vi "CameraReadJPEG.vi"(11 "IO Cluster In":T1={"Error"={"status"=FALSE, "code"=0, "source"=""}, "Encoder Calibration Values"=[22, 216], "Update Calibration"=FALSE, "JPEG Resolutions"=3, "Raw Resolutions"=1, "Image Mode"=enum."RAW Gray Scale", "FPGA Ref"=refnum} {"JPEG Resolutions" items=["160x128"=3, "320x240"=5, "640x480"=7]; "Raw Resolutions" items=["80x60"=1, "160x120"=3, "128x128"=9, "128x96"=11]}) -> (1 "New Image Data":bool, 2 "Image Data":u8[](array[numeric]) format="%02x", 3 "IO Cluster Out":T1={"Error"={"status"=FALSE, "code"=0, "source"=""}, "Encoder Calibration Values"=[22, 216], "Update Calibration"=FALSE, "JPEG Resolutions"=3, "Raw Resolutions"=1, "Image Mode"=enum."RAW Gray Scale", "FPGA Ref"=refnum} {"JPEG Resolutions" items=["160x128"=3, "320x240"=5, "640x480"=7]; "Raw Resolutions" items=["80x60"=1, "160x120"=3, "128x128"=9, "128x96"=11]}, 4 "Bytes in Buffer":u32, 5 "Image Comm Error":bool)   [LabVIEW 2019]
uses:
  JPEG Read States.ctl
  QNET MS IO Cluster.ctl
panel:
  out "Current Package":u16
  out "Picture Info Bytes":u8[](array[numeric]) format="%x"
  out "Packages":u32
  out "State":T2=enum."JPEG Picture Info"
  out "Wait for Get Picture ACK Error":bool
  out "Raw Picture Info Error":bool
  out "Bytes to Recieve":u32
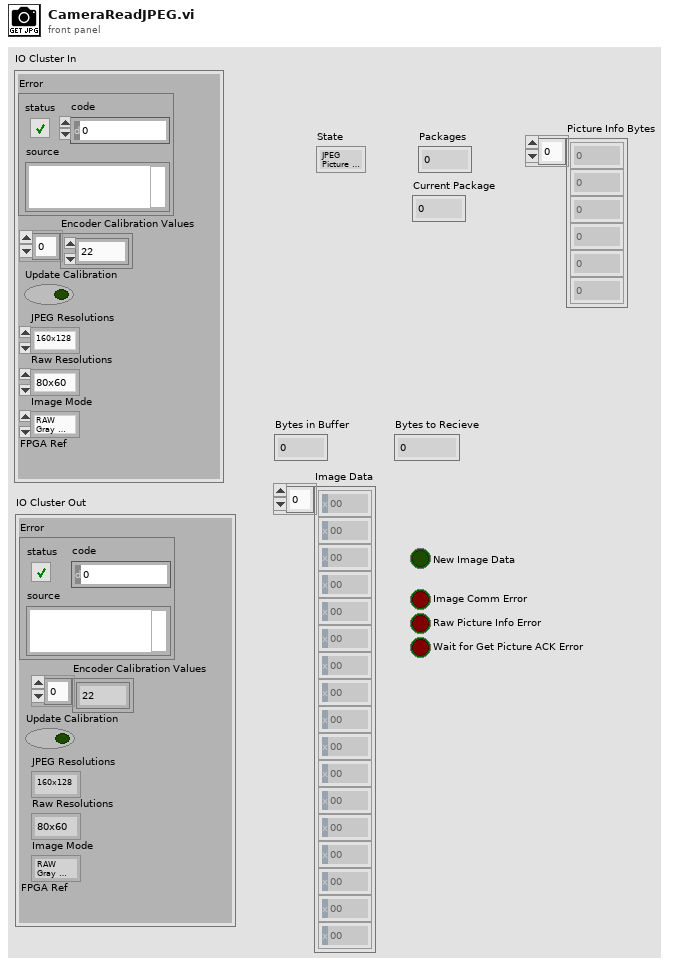
[diagram p1: front panel]
types:
  T1 = typedef "QNET MS IO Cluster.ctl" = cluster{"Error":errorcluster, "Encoder Calibration Values":i32[], "Update Calibration":bool, "JPEG Resolutions":u16, "Raw Resolutions":u16, "Image Mode":enum16{"RAW RGB", "RAW Gray Scale", "JPEG"}, "FPGA Ref":refnum<k20>}
  T2 = typedef "JPEG Read States.ctl" = enum16{"Wait for ACK", "Request Picture", "JPEG Picture Info", "Done", "Error", "Image Data"}
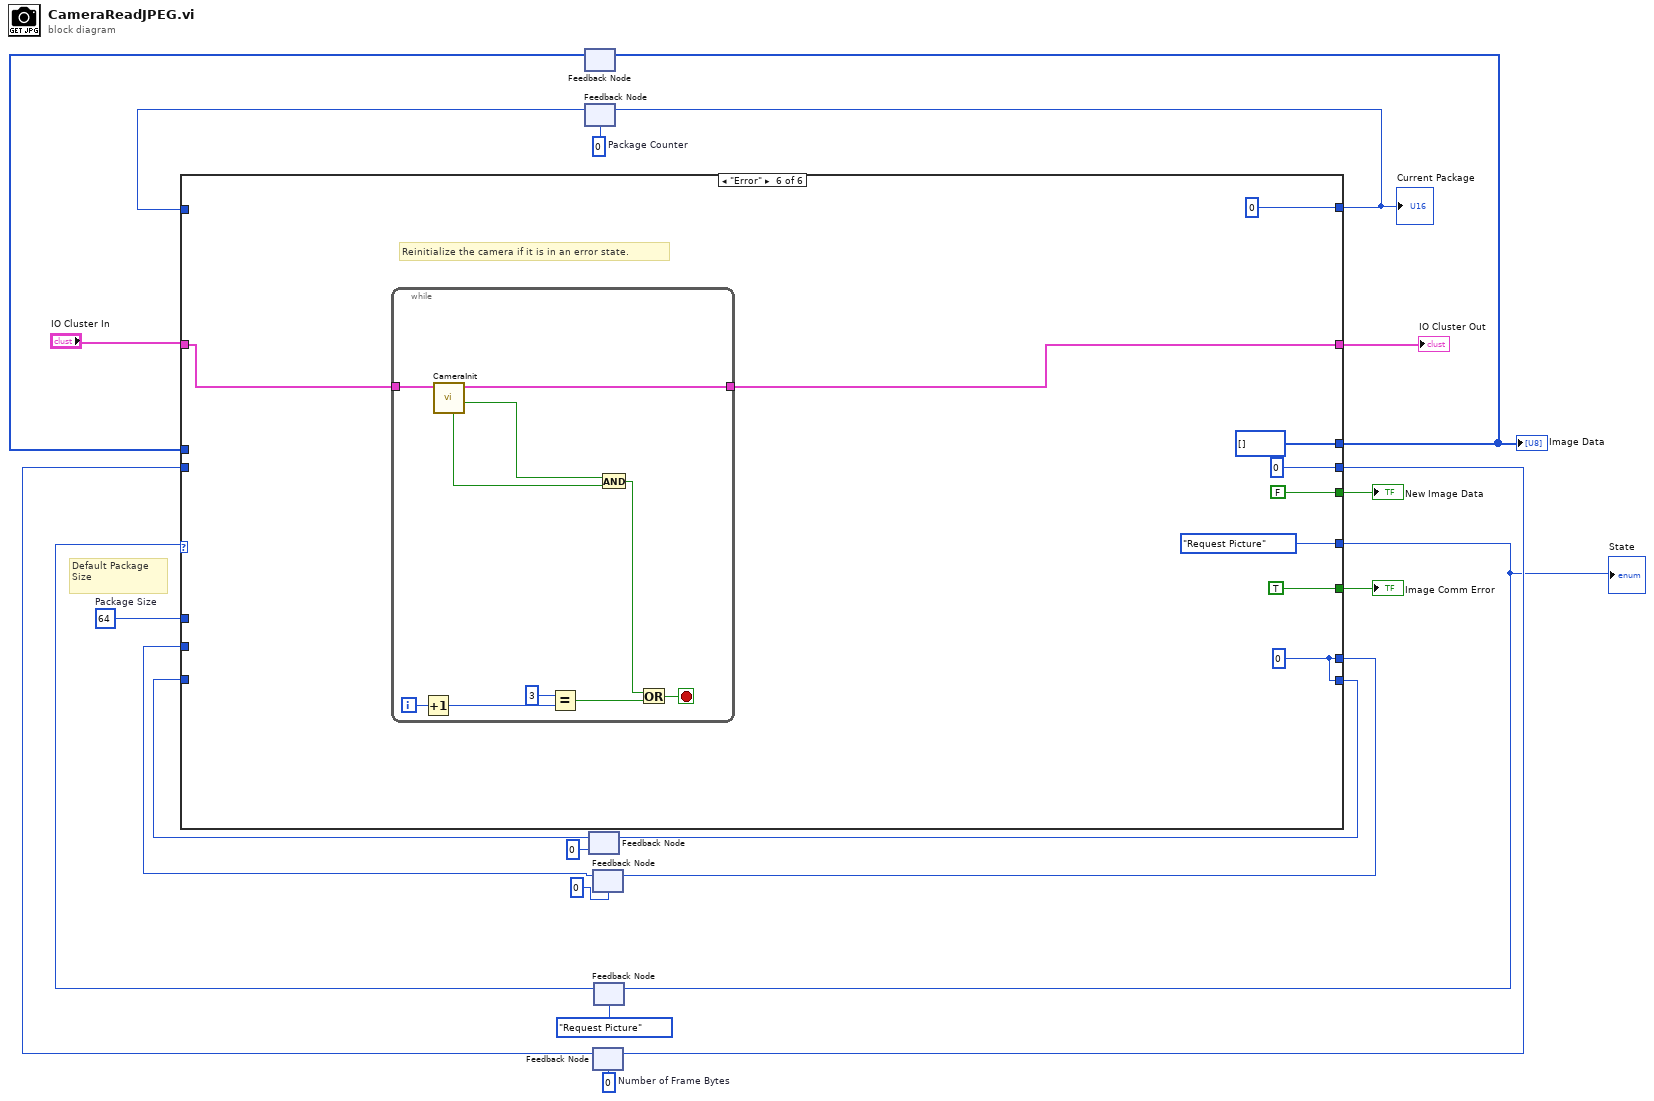
[diagram p0: block diagram]
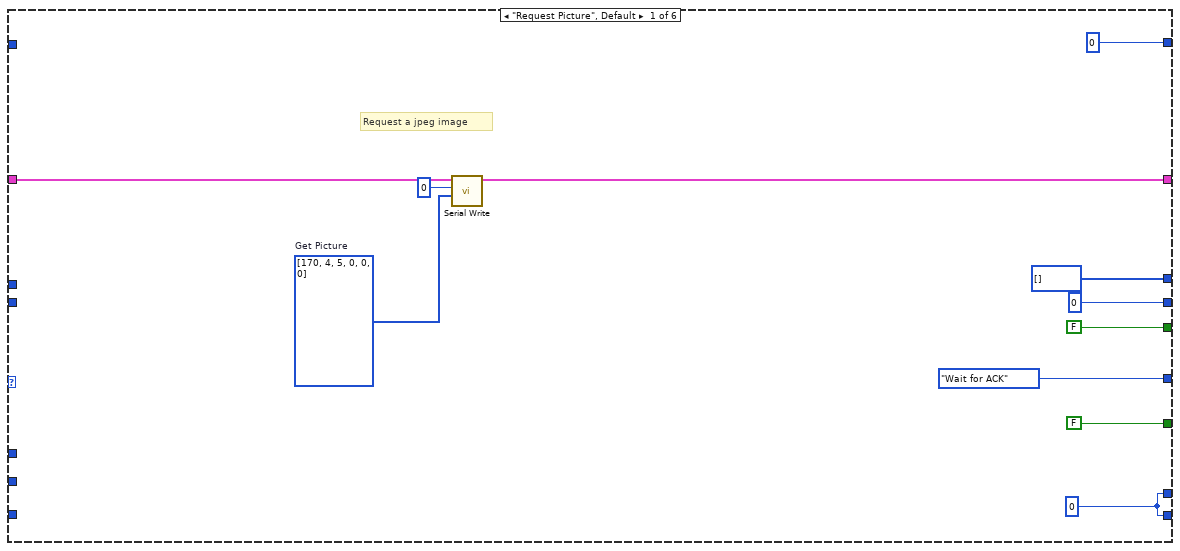
[diagram p2: hidden frame]
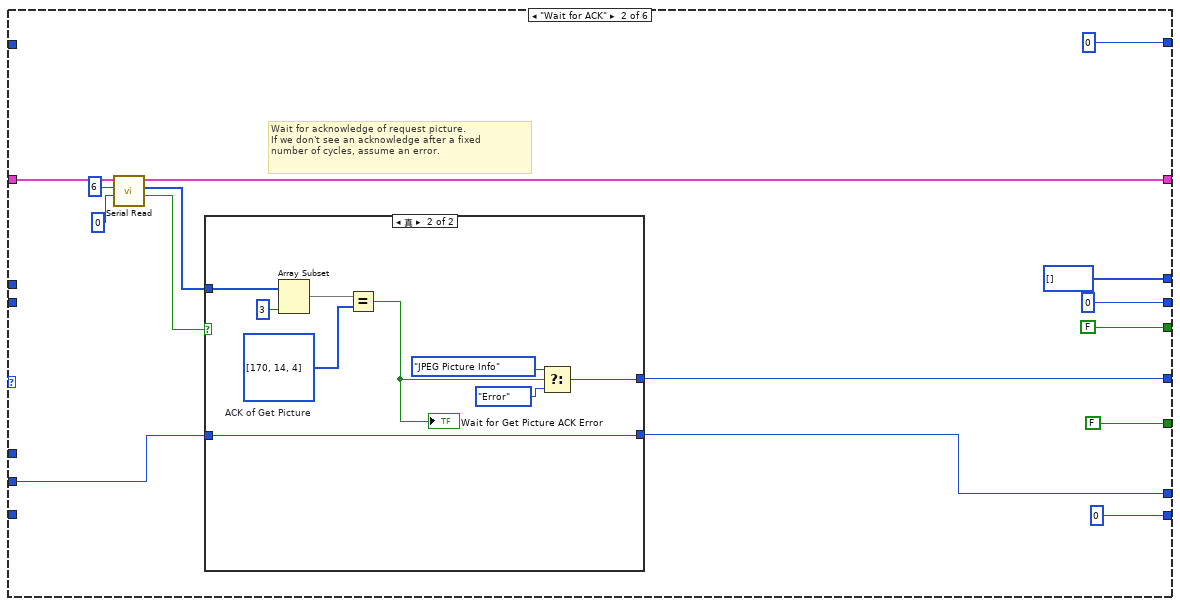
[diagram p3: hidden frame]
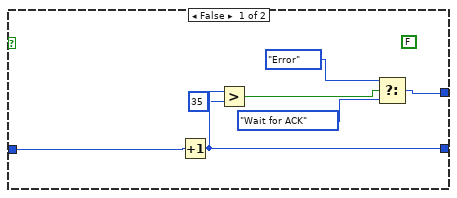
[diagram p4: hidden frame]
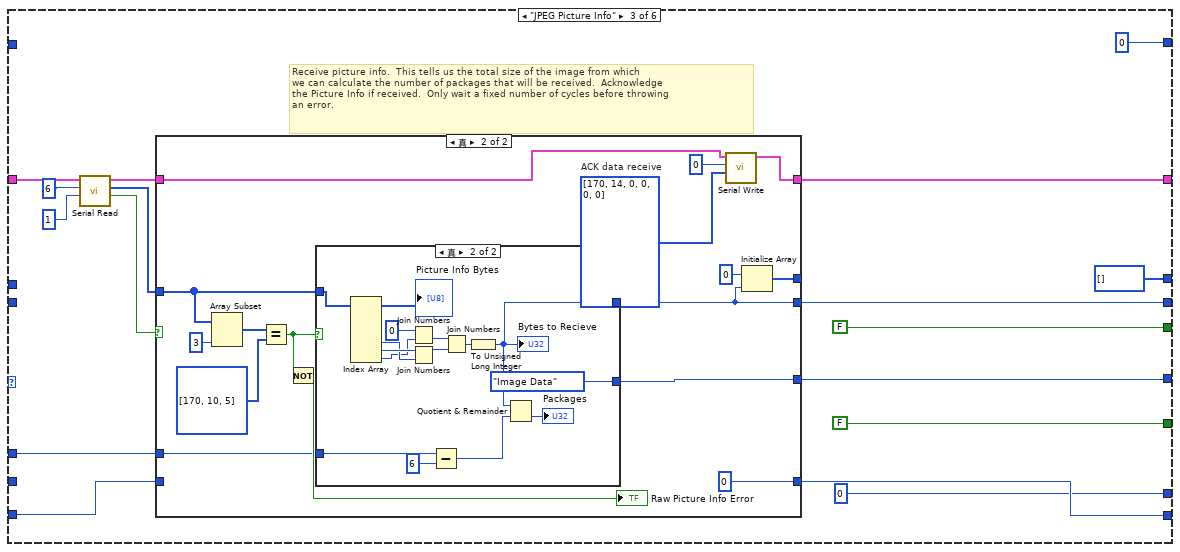
[diagram p5: hidden frame]
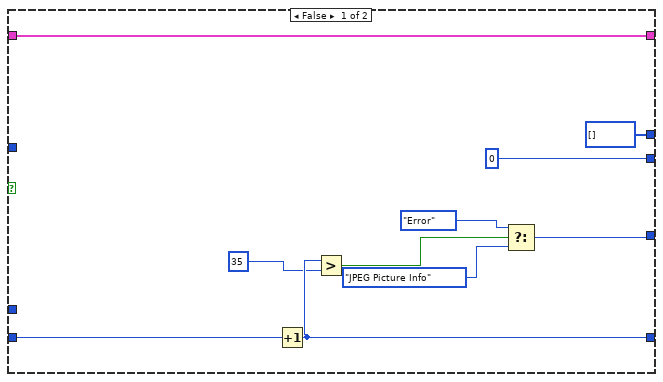
[diagram p6: hidden frame]
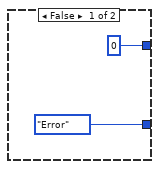
[diagram p7: hidden frame]
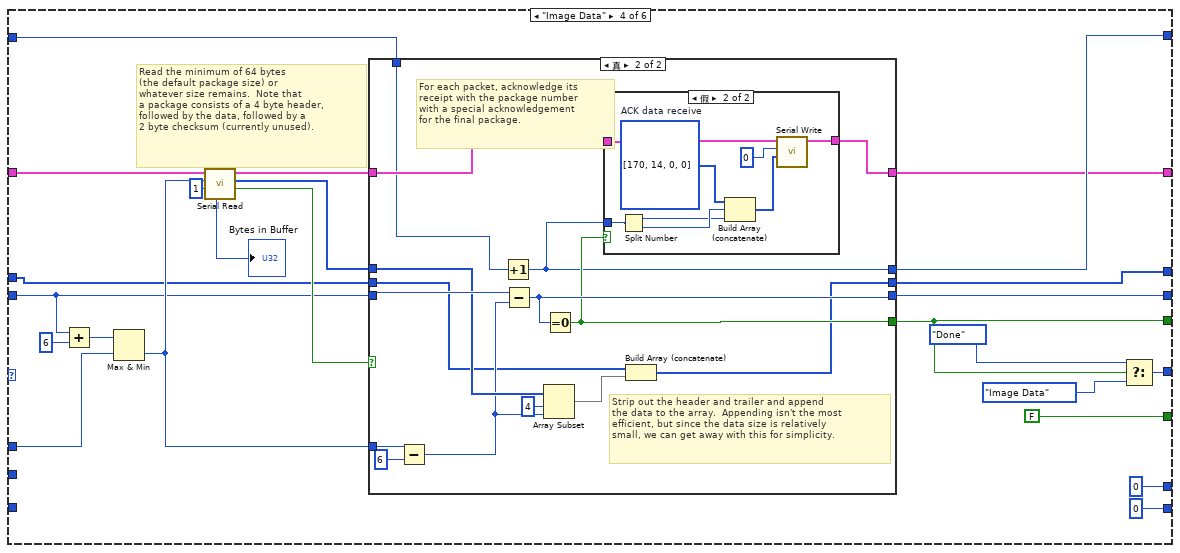
[diagram p8: hidden frame]
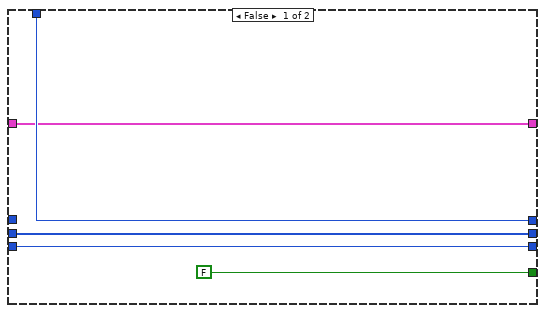
[diagram p9: hidden frame]
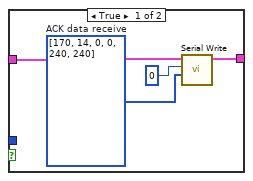
[diagram p10: hidden frame]
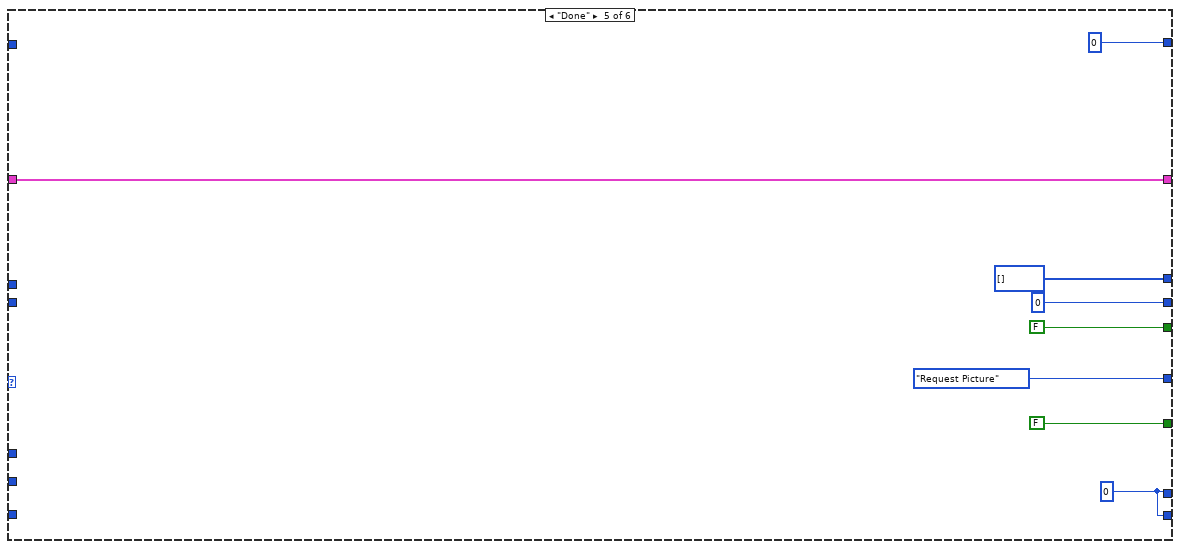
[diagram p11: hidden frame]
diagram:
  w6 = u16 0  # Package Counter
  w8 = u32 64  # Package Size
  w20 = u32 0  # Number of Frame Bytes
  # "Default Package\nSize"
  n1 = feedback #1() -> (w3:u8[])  [unwired: 1 in]
  n2 = feedback #2(w6) -> (w5:u16)
  n3 = feedback #3(0) -> (w15:i32)
  n4 = feedback #4(0) -> (w11:i32)
  n5 = feedback #5(w20) -> (w19:u32)
  n6 = feedback #6(JPEG_Read_States."Request Picture" ("Enum")) -> (w22:T2)
  n7 = case shown="\"Error\"" w22 {
    tunnel: "IO Cluster In" -> [w32 w42 w77 w146 w187 w192]
    tunnel: [JPEG_Read_States."Wait for ACK" ("Enum") w48 w81 w147 JPEG_Read_States."Request Picture" ("Enum") JPEG_Read_States."Request Picture" ("Enum")] -> w10
    tunnel: [u32 0 ("Number of Frame Bytes") u32 0 w80 w137 u32 0 ("Number of Frame Bytes") u32 0 ("Number of Frame Bytes")] -> w21
    tunnel: w19 -> [_ _ _ w133 _ _]
    tunnel: [w29 w35 w66 w128 w187 w191] -> w1
    tunnel: [u8[] [] ("Data") u8[] [] ("Data") u8[] [] ("Data") w126 u8[] [] ("Data") u8[] [] ("Data")] -> w4
    tunnel: [FALSE ("Data Valid") FALSE ("Data Valid") FALSE ("Data Valid") w130 FALSE ("Data Valid") FALSE ("Data Valid")] -> w18
    tunnel: [FALSE FALSE FALSE FALSE FALSE TRUE] -> w17
    tunnel: [w25 0 w72 0 w182 w193] -> w16
    tunnel: w15 -> [_ _ w71 _ _ _]
    tunnel: [w25 w36 0 0 w182 w193] -> w12
    tunnel: w11 -> [_ w37 _ _ _ _]
    tunnel: w8 -> [_ _ w69 w138 _ _]
    tunnel: [u16 0 u16 0 u16 0 w135 u16 0 u16 0] -> w7
    tunnel: w5 -> [_ _ _ w136 _ _]
    tunnel: w3 -> [_ _ _ w127 _ _]
    frame "Request Picture", Default {
      w25 = 0
      w31 = u8[] [170, 4, 5, 0, 0, 0]  # Get Picture
      # "Request a jpeg image"
      n8 = call "Serial Write.vi"("Array"=w31, "Timeout (ms)"=0, "IO Cluster In"=w32) -> ("IO Cluster Out"=w29:T1)  [unwired: 8 in]
    }
    frame "Wait for ACK" {
      # "Wait for acknowledge of request picture.\nIf we don't see an acknowledge after a fixed\nnumber of cycles, assume an error."
      n9 = call "Serial Read.vi"("Timeout (ms)"=0, "Number of Bytes to Read"=u32 6 ("bytes to read"), "IO Cluster In"=w42) -> ("Data Valid"=w44:bool, "Data"=w43:u8[], "IO Cluster Out"=w35:T1)  [unwired: 4 in, 2 out]
      n10 = case shown="真" w44 {
        tunnel: w43 -> [_ w64]
        tunnel: [w52 w60] -> w48
        tunnel: w37 -> [w55 w58]
        tunnel: [w54 w58] -> w36
        frame False {
          (unwired) FALSE
          n11 = Increment(x=w55) -> (x+1=w54:i32)
          n12 = Greater?(x=w54, y=35) -> (0:w51:bool)
          n13 = Select(t=JPEG_Read_States."Error" ("Enum"), s=w51, f=JPEG_Read_States."Wait for ACK" ("Enum")) -> (s? t:f=w52:T2)
        }
        frame True {
          w62 = u8[] [170, 14, 4]  # ACK of Get Picture
          n14 = Array Subset(array=w64, length=3) -> (w57:u8[])  [unwired: 1 in]
          n15 = Equal?(x=w57, y=w62) -> (x = y?=w59:bool)
          "Wait for Get Picture ACK Error" <- w59
          n16 = Select(t=JPEG_Read_States."JPEG Picture Info" ("Enum"), s=w59, f=JPEG_Read_States."Error" ("Enum")) -> (s? t:f=w60:T2)
        }
      }
    }
    frame "JPEG Picture Info" {
      # "Receive picture info.  This tells us the total size of the image from which\nwe can calculate the number of packages that will be received.  Acknowledge\nthe Picture Info if received.  Only wait a fixed number of cycles before throwing\nan error."
      n17 = call "Serial Read.vi"("Timeout (ms)"=1, "Number of Bytes to Read"=u32 6 ("bytes to read"), "IO Cluster In"=w77) -> ("Data Valid"=w79:bool, "Data"=w78:u8[], "IO Cluster Out"=w67:T1)  [unwired: 4 in, 2 out]
      n18 = case shown="真" w79 {
        tunnel: w78 -> [_ w100]
        tunnel: [w87 w104] -> w81
        tunnel: [u32 0 w93] -> w80
        tunnel: [w89 0] -> w72
        tunnel: w71 -> [w90 _]
        tunnel: w69 -> [_ w99]
        tunnel: w67 -> [w83 w96]
        tunnel: [w83 w95] -> w66
        tunnel: [u8[] [] w92] -> _
        frame False {
          n19 = Increment(x=w90) -> (x+1=w89:i32)
          n20 = Greater?(x=w89, y=35) -> (0:w86:bool)
          n21 = Select(t=JPEG_Read_States."Error" ("Enum"), s=w86, f=JPEG_Read_States."JPEG Picture Info" ("Enum")) -> (s? t:f=w87:T2)
        }
        frame True {
          w98 = u8[] [170, 14, 0, 0, 0, 0]  # ACK data receive
          n22 = Array Subset(array=w100, length=3) -> (w106:u8[])  [unwired: 1 in]
          n23 = Equal?(x=w106, y=u8[] [170, 10, 5]) -> (x = y?=w102:bool)
          n24 = Not(x=w102) -> (.not. x?=→"Raw Picture Info Error":bool)
          n25 = case shown="真" w102 {
            tunnel: [JPEG_Read_States."Error" ("Enum") JPEG_Read_States."Image Data" ("Enum")] -> w104
            tunnel: w100 -> [_ w123]
            tunnel: [u32 0 w116] -> w93
            tunnel: w99 -> [_ w112]
            frame False {
            }
            frame True {
              n26 = Index Array(array=w123) -> (element #4=w114:u8, element #5=w122:u8, element #6=w113:u8)  [unwired: 6 in, 3 out]
              n27 = Join Numbers(hi=u8 0, lo=w113) -> ((hi.lo)=w120:u16)
              n28 = Join Numbers(hi=w122, lo=w114) -> ((hi.lo)=w119:u16)
              n29 = Subtract(x=w112, y=u32 6) -> (x-y=w111:u32)
              n30 = Join Numbers(hi=w120, lo=w119) -> ((hi.lo)=w118:u32)
              n31 = To Unsigned Long Integer(number=w118) -> (unsigned 32bit integer=w116:u32)
              "Bytes to Recieve" <- w116
              n32 = Quotient & Remainder(x=w116, y=w111) -> (floor(x/y)=→"Packages":u32)  [unwired: 1 out]
              "Picture Info Bytes" <- w123
            }
          }
          n33 = call "Serial Write.vi"("Array"=w98, "Timeout (ms)"=0, "IO Cluster In"=w96) -> ("IO Cluster Out"=w95:T1)  [unwired: 8 in]
          n34 = Initialize Array(u8 0 ("element"), w93) -> (w92:u8[])
        }
      }
    }
    frame "Image Data" {
      # "Read the minimum of 64 bytes \n(the default package size) or \nwhatever size remains.  Note that\na package consists of a 4 byte header,\nfollowed by the data, followed by a\n2 byte checksum (currently unused)."
      n35 = Add(x=w133, y=u32 6) -> (x+y=w132:u32)
      n36 = Max & Min(x=w132, y=w138) -> (min(x,y)=w134:u32)  [unwired: 1 out]
      n37 = call "Serial Read.vi"("Timeout (ms)"=1, "Number of Bytes to Read"=w134, "IO Cluster In"=w146) -> ("Data Valid"=w140:bool, "Data"=w139:u8[], "IO Cluster Out"=w129:T1, "Bytes in Buffer"=→"Bytes in Buffer":u32)  [unwired: 4 in, 1 out]
      n38 = case shown="真" w140 {
        tunnel: w139 -> [_ w158]
        tunnel: w133 -> [w152 w165]
        tunnel: w134 -> [_ w167]
        tunnel: [w152 w164] -> w137
        tunnel: w136 -> [w151 w161]
        tunnel: [w151 w159] -> w135
        tunnel: [FALSE w160] -> w130
        tunnel: w129 -> [w149 w163]
        tunnel: [w149 w162] -> w128
        tunnel: w127 -> [w148 w154]
        tunnel: [w148 w153] -> w126
        frame False {
        }
        frame True {
          # "Strip out the header and trailer and append\nthe data to the array.  Appending isn't the most\nefficient, but since the data size is relatively\nsmall, we can get away with this for simplicity."
          # "For each packet, acknowledge its\nreceipt with the package number\nwith a special acknowledgement\nfor the final package."
          n39 = Subtract(x=w167, y=u32 6) -> (x-y=w156:u32)
          n40 = Increment(x=w161) -> (x+1=w159:u16)
          n41 = Subtract(x=w165, y=w156) -> (x-y=w164:u32)
          n42 = Array Subset(array=w158, index=4, length=w156) -> (w155:u8[])
          n43 = Equal To 0?(x=w164) -> (x = 0?=w160:bool)
          n44 = case shown="假" w160 {
            tunnel: w163 -> [w169 w178]
            tunnel: [w168 w177] -> w162
            tunnel: w159 -> [_ w174]
            frame True {
              w170 = u8[] [170, 14, 0, 0, 240, 240]  # ACK data receive
              n45 = call "Serial Write.vi"("Array"=w170, "Timeout (ms)"=0, "IO Cluster In"=w169) -> ("IO Cluster Out"=w168:T1)  [unwired: 8 in]
            }
            frame False {
              w176 = u8[] [170, 14, 0, 0]  # ACK data receive
              n46 = Split Number(x=w174) -> (hi(x)=w172:u8, lo(x)=w173:u8)
              n47 = Build Array (concatenate)(w176, w173, w172) -> (w175:u8[])
              n48 = call "Serial Write.vi"("Array"=w175, "Timeout (ms)"=0, "IO Cluster In"=w178) -> ("IO Cluster Out"=w177:T1)  [unwired: 8 in]
            }
          }
          n49 = Build Array (concatenate)(w154, w155) -> (w153:u8[])
        }
      }
      n50 = Select(t=JPEG_Read_States."Done" ("Enum"), s=w130, f=JPEG_Read_States."Image Data" ("Enum")) -> (s? t:f=w147:T2)
    }
    frame "Done" {
      w182 = 0
    }
    frame "Error" {
      w193 = 0
      # "Reinitialize the camera if it is in an error state."
      n51 = while {
        tunnel: w192 -> [w201]
        tunnel: [w200] -> w191
        i -> [w206]
        stop <- w203 stop-if-true
        n52 = Increment(x=w206) -> (x+1=w202:i32)
        n53 = call "CameraInit.vi"("IO Cluster In"=w201) -> ("Sync Complete"=w199:bool, "IO Cluster Out"=w200:T1, "Camera Configured"=w198:bool)  [unwired: 7 in, 1 out]
        n54 = Equal?(x=3, y=w202) -> (x = y?=w204:bool)
        n55 = And(x=w199, y=w198) -> (x .and. y?=w197:bool)
        n56 = Or(x=w197, y=w204) -> (x .or. y?=w203:bool)
      }
    }
  }
  "New Image Data" <- w18
  "Image Data" <- w4
  "Image Comm Error" <- w17
  "State" <- w10
  "Current Package" <- w7
  "IO Cluster Out" <- w1
  n57 = feedback-in #1(w4) -> ()
  n58 = feedback-in #2(w7) -> ()
  n59 = feedback-in #3(w16) -> ()
  n60 = feedback-in #4(w12) -> ()
  n61 = feedback-in #5(w21) -> ()
  n62 = feedback-in #6(w10) -> ()
